vi "模块参数配置.vi"(9 "路径":path, 10 "历史中心参数2":T2={"IP地址"="192.168.1.1", "工作模式"=48, "连接协议"=48, "本机号码"="13806871122", "短信监控中心号码1"="13800577500", "监听时间"=0, "心跳间隔"=0, "重启时间(分)"=0, "C/S关系"=48, "DNS域名"="", "APN接入点"="", "报头使能"=48, "波特率"=45060, "短信目标号码1 "="", "短信目标号码2"="", "短信监控中心号码2"="", "信号检测使能"=48, "控制方式"=48, "端口号"=5070, "连接方式"=48} {"连接方式" items=["固定IP"=48, "域名解析"=49]; "控制方式" items=["软件控制"=48, "EN控制"=49]; "信号检测使能" items=["不检测"=48, "检测"=49]; "波特率" items=["1200"=45060, "2400"=24585, "4800"=49170, "9600"=32805, "19200"=75]; "报头使能" items=["上传"=48, "不上传"=49]; "C/S关系" items=["客服端"=48, "服务端"=49]; "连接协议" items=["TCP协议"=48, "UDP协议"=49]; "工作模式" items=["GPRS模式"=48, "短信模式"=49]}, 11 "历史中心参数1":T2={"IP地址"="192.168.1.1", "工作模式"=48, "连接协议"=48, "本机号码"="13806871122", "短信监控中心号码1"="13800577500", "监听时间"=0, "心跳间隔"=0, "重启时间(分)"=0, "C/S关系"=48, "DNS域名"="", "APN接入点"="", "报头使能"=48, "波特率"=45060, "短信目标号码1 "="", "短信目标号码2"="", "短信监控中心号码2"="", "信号检测使能"=48, "控制方式"=48, "端口号"=5070, "连接方式"=48} {"连接方式" items=["固定IP"=48, "域名解析"=49]; "控制方式" items=["软件控制"=48, "EN控制"=49]; "信号检测使能" items=["不检测"=48, "检测"=49]; "波特率" items=["1200"=45060, "2400"=24585, "4800"=49170, "9600"=32805, "19200"=75]; "报头使能" items=["上传"=48, "不上传"=49]; "C/S关系" items=["客服端"=48, "服务端"=49]; "连接协议" items=["TCP协议"=48, "UDP协议"=49]; "工作模式" items=["GPRS模式"=48, "短信模式"=49]}) -> ()   [LabVIEW 2015]
uses:
  <vilib>/Utility/config.llb/Config Data RefNum.ctl
  <vilib>/Utility/config.llb/Write Key (String).vi
  <vilib>/Utility/config.llb/NI_LVConfig.lvlib
panel:
  out "输出配置文件":T1 caption="refnum out"
  out "保存参数数组":bool[](array[boolean])
  out "读参数数组":bool[](array[boolean])
  out "写参数数组":bool[](array[boolean])
  out "复制数组":bool[](array[boolean])
  in  "》2":bool
  in  "》1":bool
  in  "模块中心参数2":T2={"IP地址"="192.168.1.1", "工作模式"=48, "连接协议"=48, "本机号码"="13806871122", "短信监控中心号码1"="13800577500", "监听时间"=0, "心跳间隔"=0, "重启时间(分)"=0, "C/S关系"=48, "DNS域名"="", "APN接入点"="", "报头使能"=48, "波特率"=45060, "短信目标号码1 "="", "短信目标号码2"="", "短信监控中心号码2"="", "信号检测使能"=48, "控制方式"=48, "端口号"=5070, "连接方式"=48} {"连接方式" items=["固定IP"=48, "域名解析"=49]; "控制方式" items=["软件控制"=48, "EN控制"=49]; "信号检测使能" items=["不检测"=48, "检测"=49]; "波特率" items=["1200"=45060, "2400"=24585, "4800"=49170, "9600"=32805, "19200"=75]; "报头使能" items=["上传"=48, "不上传"=49]; "C/S关系" items=["客服端"=48, "服务端"=49]; "连接协议" items=["TCP协议"=48, "UDP协议"=49]; "工作模式" items=["GPRS模式"=48, "短信模式"=49]}
  in  "模块中心参数1":T2={"IP地址"="192.168.1.1", "工作模式"=48, "连接协议"=48, "本机号码"="13806871122", "短信监控中心号码1"="13800577500", "监听时间"=0, "心跳间隔"=0, "重启时间(分)"=0, "C/S关系"=48, "DNS域名"="", "APN接入点"="", "报头使能"=48, "波特率"=45060, "短信目标号码1 "="", "短信目标号码2"="", "短信监控中心号码2"="", "信号检测使能"=48, "控制方式"=48, "端口号"=5070, "连接方式"=48} {"连接方式" items=["固定IP"=48, "域名解析"=49]; "控制方式" items=["软件控制"=48, "EN控制"=49]; "信号检测使能" items=["不检测"=48, "检测"=49]; "波特率" items=["1200"=45060, "2400"=24585, "4800"=49170, "9600"=32805, "19200"=75]; "报头使能" items=["上传"=48, "不上传"=49]; "C/S关系" items=["客服端"=48, "服务端"=49]; "连接协议" items=["TCP协议"=48, "UDP协议"=49]; "工作模式" items=["GPRS模式"=48, "短信模式"=49]}
  in  "写入模块参数二":bool
  in  "写入模块参数一":bool
  in  "保存历史参数二":bool
  in  "保存历史参数一":bool
  in  "获取模块参数二":bool
  in  "获取模块参数一":bool
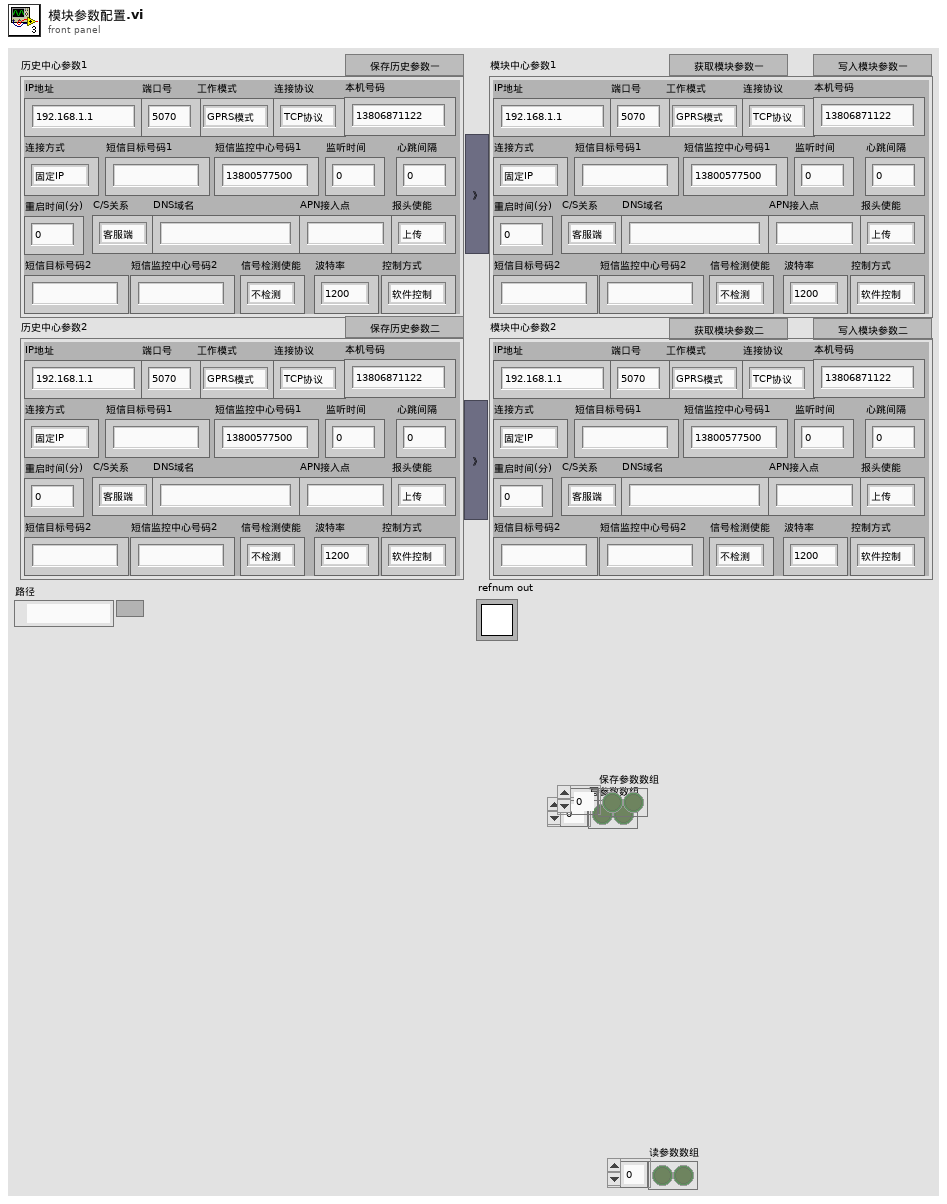
[diagram p1: front panel]
types:
  T1 = typedef "NI_LVConfig.lvlib/Config Data RefNum.ctl" = refnum<k1>
  T2 = typedef "GPRS参数DW02.ctl" = cluster{"IP地址":string, "工作模式":u16, "连接协议":u16, "本机号码":string, "短信监控中心号码1":string, "监听时间":u16, "心跳间隔":u16, "重启时间(分)":u16, "C/S关系":u16, "DNS域名":string, "APN接入点":string, "报头使能":u16, "波特率":u16, "短信目标号码1 ":string, "短信目标号码2":string, "短信监控中心号码2":string, "信号检测使能":u16, "控制方式":u16, "端口号":u16, "连接方式":u16}
  T3 = typedef "模块参数配置状态机状态(枚举).ctl" = enum16{"初始化", "加载参数", "等待按键", "写参数", "读参数", "拷贝参数", "保存参数", "退出"}
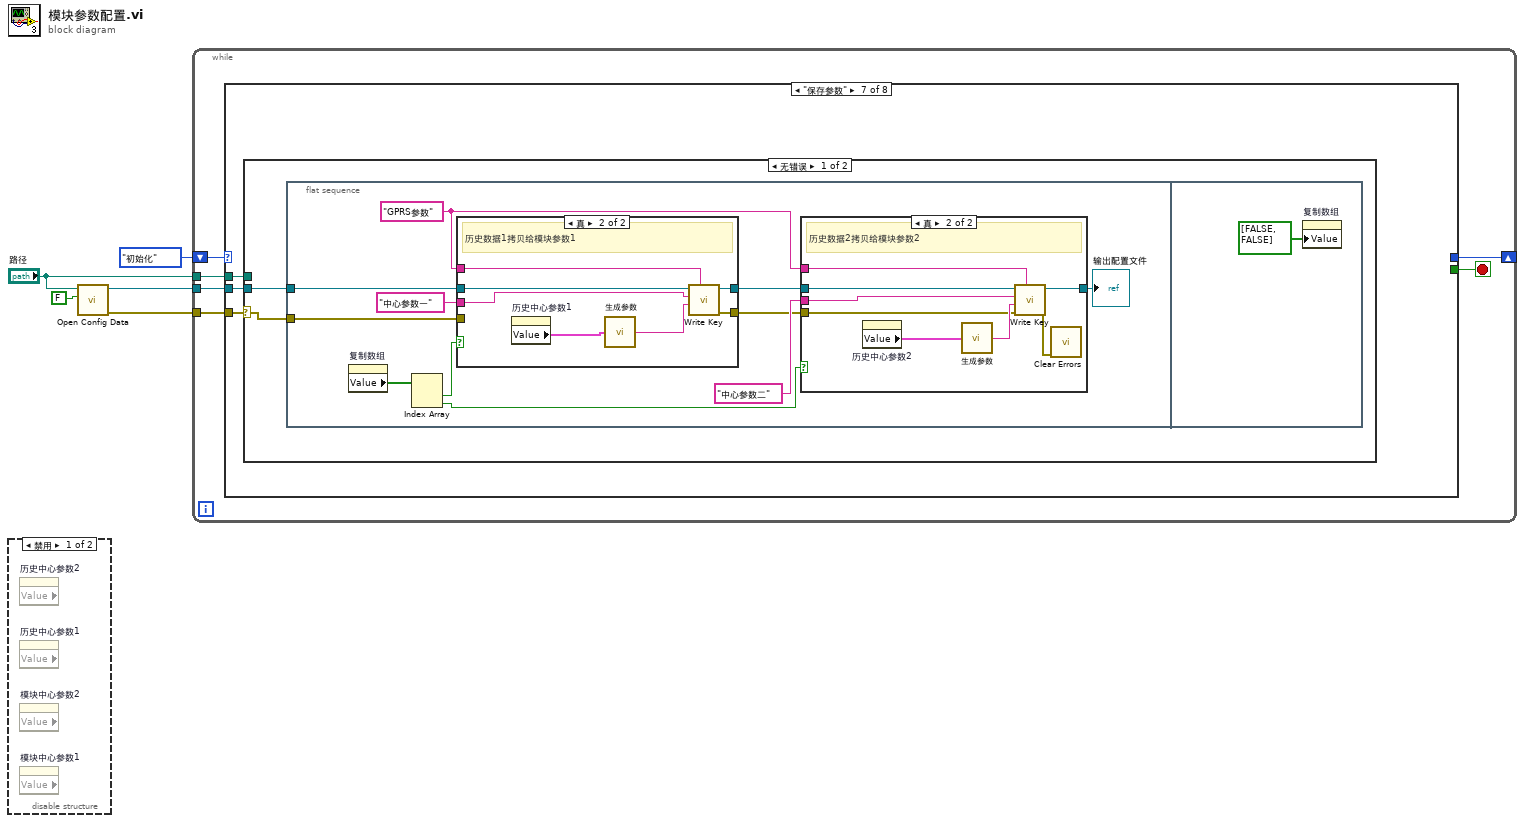
[diagram p0: block diagram]
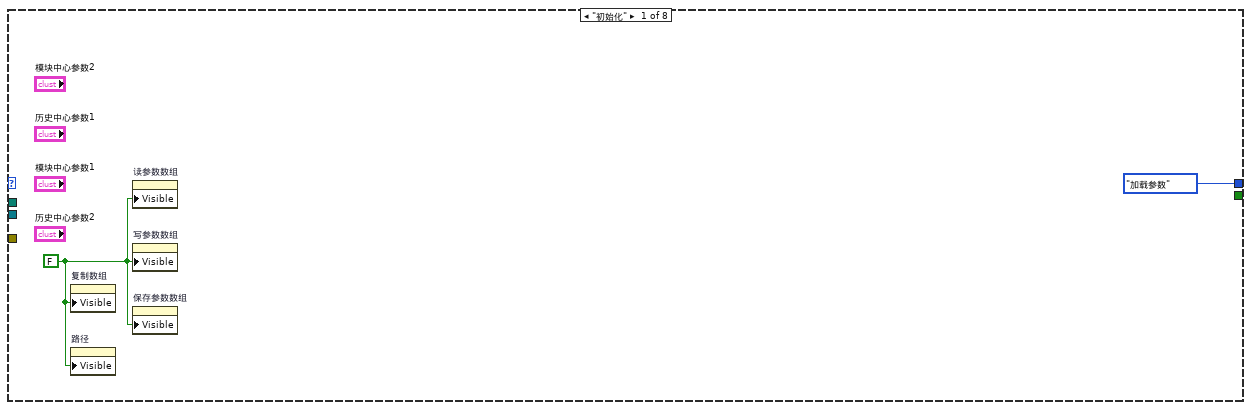
[diagram p3: hidden frame]
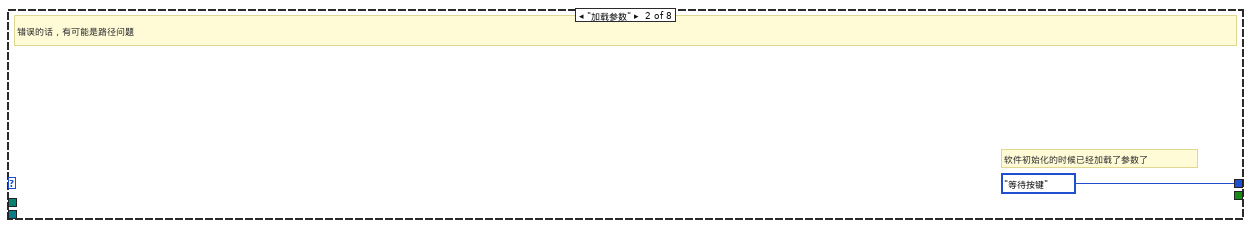
[diagram p4: hidden frame]
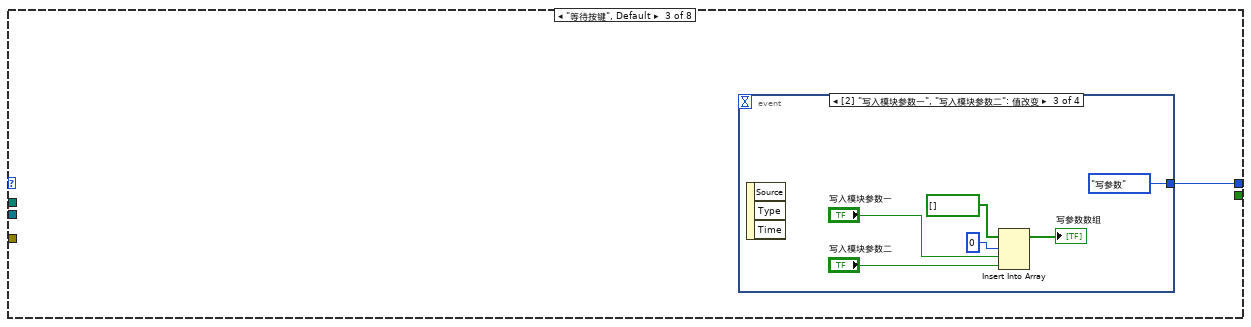
[diagram p5: hidden frame]
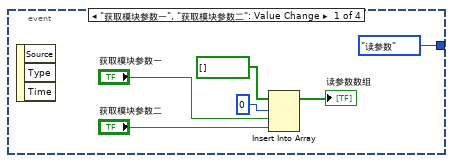
[diagram p6: hidden frame]
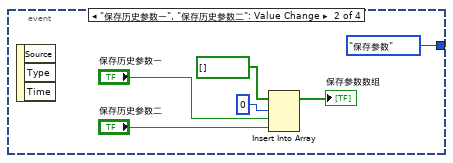
[diagram p7: hidden frame]
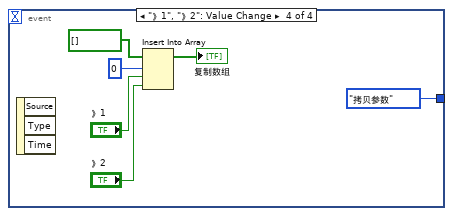
[diagram p8: hidden frame]
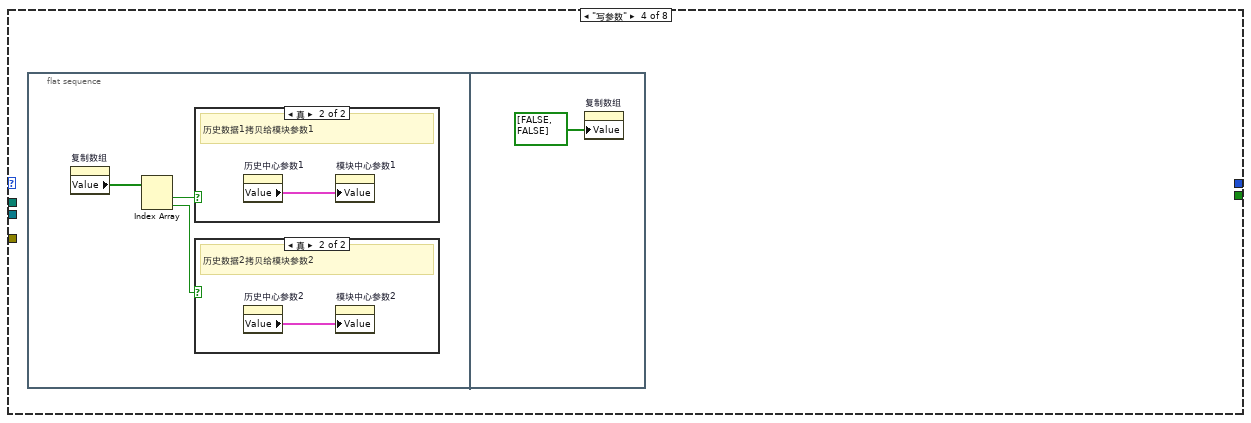
[diagram p9: hidden frame]
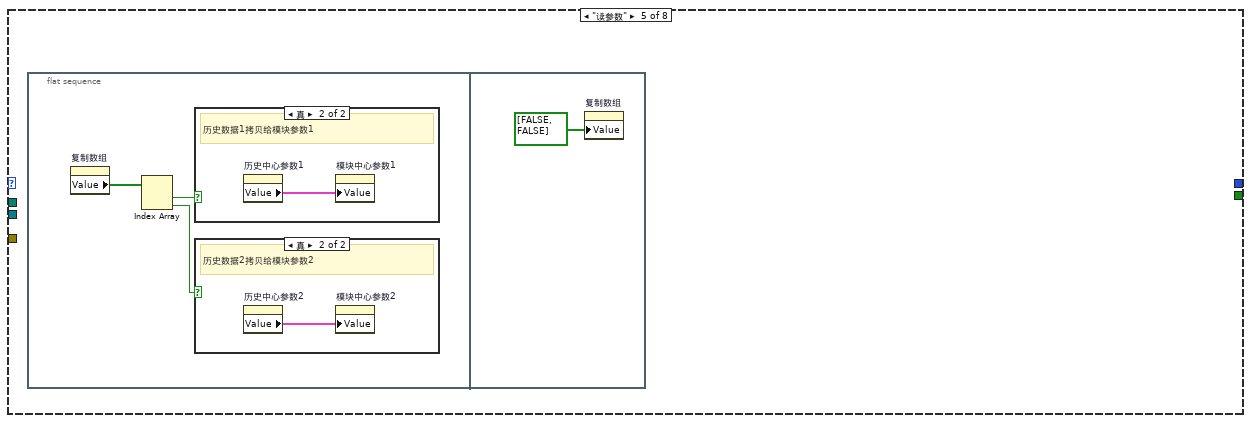
[diagram p12: hidden frame]
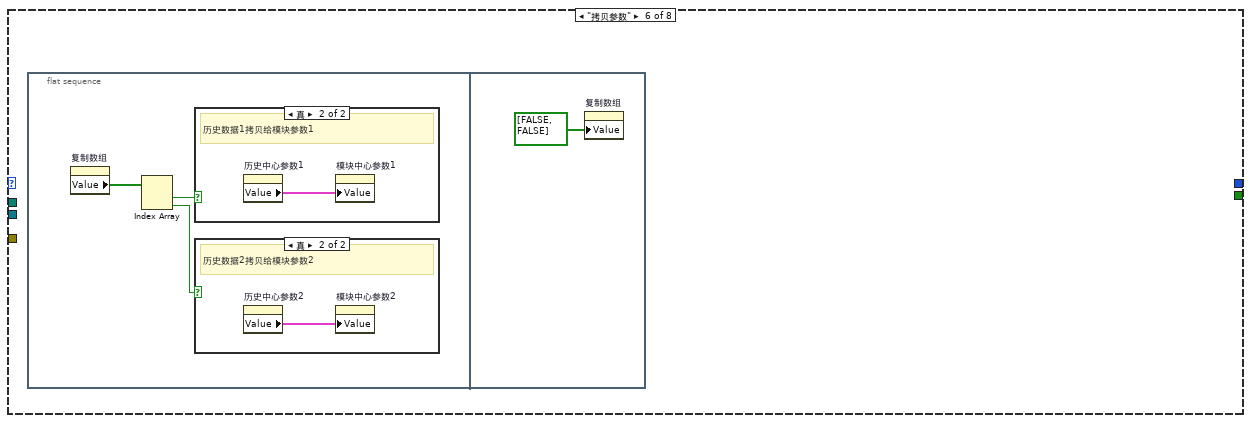
[diagram p15: hidden frame]
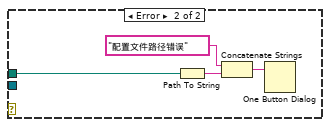
[diagram p20: hidden frame]
diagram:
  n1 = disable-structure shown="禁用" {
    frame Disabled {
      n2 = property on="历史中心参数2" class="Clust (严格)" props=["Value"]() -> ()  [unwired: 2 in, 3 out]
      n3 = property on="历史中心参数1" class="Clust (严格)" props=["Value"]() -> ()  [unwired: 2 in, 3 out]
      n4 = property on="模块中心参数2" class="Clust (严格)" props=["Value"]() -> ()  [unwired: 2 in, 3 out]
      n5 = property on="模块中心参数1" class="Clust (严格)" props=["Value"]() -> ()  [unwired: 2 in, 3 out]
    }
    frame Enabled {
    }
  }
  n6 = call <vilib>:"Open Config Data.vi"("create file if necessary (T)"=FALSE, "configuration file path"="路径") -> ("error out"=w2:errorcluster, "refnum"=w3:T1)  [unwired: 7 in, 1 out]
  n7 = while {
    shift-right: [w10] -> _
    shift-left: 模块参数配置状态机状态(枚举)."初始化" -> [w9]
    tunnel: w3 -> [w8]
    tunnel: w2 -> [w7]
    tunnel: "路径" -> [w6]
    stop <- w11 stop-if-true
    n8 = case shown="\"保存参数\"" w9 {
      tunnel: [_ _ _ _ _ _ _ TRUE] -> w11
      tunnel: [模块参数配置状态机状态(枚举)."加载参数" 模块参数配置状态机状态(枚举)."等待按键" w15 _ _ _ _ _] -> w10
      tunnel: w8 -> [_ _ _ _ _ _ w60 _]
      tunnel: w7 -> [_ _ _ _ _ _ w59 _]
      tunnel: w6 -> [_ _ _ _ _ _ w58 _]
      frame "初始化" {
        w12 = FALSE ("可见")
        n9 = property on="复制数组" class="Arr (严格)"("Visible"=w12) -> ()  [unwired: 2 in, 2 out]
        n10 = property on="路径" class="Path"("Visible"=w12) -> ()  [unwired: 2 in, 2 out]
        n11 = property on="读参数数组" class="Arr (严格)"("Visible"=w12) -> ()  [unwired: 2 in, 2 out]
        n12 = property on="写参数数组" class="Arr (严格)"("Visible"=w12) -> ()  [unwired: 2 in, 2 out]
        n13 = property on="保存参数数组" class="Arr (严格)"("Visible"=w12) -> ()  [unwired: 2 in, 2 out]
      }
      frame "加载参数" {
        # "软件初始化的时候已经加载了参数了"
        # "错误的话，有可能是路径问题"
      }
      frame "等待按键", Default {
        n14 = event shown="[2] \"写入模块参数一\", \"写入模块参数二\": 值改变" {
          selector: _ -> [_ _ _ _]
          dyn-events: _ -> [_ _ _ _]
          timeout: _ -> [_ _ _ _]
          tunnel: [模块参数配置状态机状态(枚举)."读参数" 模块参数配置状态机状态(枚举)."保存参数" 模块参数配置状态机状态(枚举)."写参数" 模块参数配置状态机状态(枚举)."拷贝参数"] -> w15
          event "获取模块参数一", "获取模块参数二": Value Change {
            n15 = event-data() -> ()  [unwired: 1 in, 3 out]
            n16 = Insert Into Array(array=bool[] [] ("数组"), index=0 ("索引"), new element #1="获取模块参数一", new element #2="获取模块参数二") -> (→"读参数数组":bool[])
          }
          event "保存历史参数一", "保存历史参数二": Value Change {
            n17 = event-data() -> ()  [unwired: 1 in, 3 out]
            n18 = Insert Into Array(array=bool[] [] ("数组"), index=0 ("索引"), new element #1="保存历史参数一", new element #2="保存历史参数二") -> (→"保存参数数组":bool[])
          }
          event "写入模块参数一", "写入模块参数二": Value Change {
            n19 = event-data() -> ()  [unwired: 1 in, 3 out]
            n20 = Insert Into Array(array=bool[] [] ("数组"), index=0 ("索引"), new element #1="写入模块参数一", new element #2="写入模块参数二") -> (→"写参数数组":bool[])
          }
          event "》1", "》2": Value Change {
            n21 = event-data() -> ()  [unwired: 1 in, 3 out]
            n22 = Insert Into Array(array=bool[] [] ("数组"), index=0 ("索引"), new element #1="》1", new element #2="》2") -> (→"复制数组":bool[])
          }
        }
      }
      frame "写参数" {
        n23 = flat-sequence {
          frame #0 {
            n24 = property on="复制数组" class="Arr (严格)"() -> ("Value"=w42:bool[])  [unwired: 2 in, 2 out]
            n25 = Index Array(array=w42) -> (element #1=w41:bool, element #2=w40:bool)  [unwired: 2 in]
            n26 = case shown="真" w41 {
              frame False {
              }
              frame True {
                # "历史数据1拷贝给模块参数1"
                n27 = property on="历史中心参数1" class="Clust (严格)"() -> ("Value"=w44:T2)  [unwired: 2 in, 2 out]
                n28 = property on="模块中心参数1" class="Clust (严格)"("Value"=w44) -> ()  [unwired: 2 in, 2 out]
              }
            }
            n29 = case shown="真" w40 {
              frame False {
              }
              frame True {
                # "历史数据2拷贝给模块参数2"
                n30 = property on="历史中心参数2" class="Clust (严格)"() -> ("Value"=w43:T2)  [unwired: 2 in, 2 out]
                n31 = property on="模块中心参数2" class="Clust (严格)"("Value"=w43) -> ()  [unwired: 2 in, 2 out]
              }
            }
          }
          frame #1 {
            n32 = property on="复制数组" class="Arr (严格)"("Value"=bool[] [FALSE, FALSE] ("复制数组")) -> ()  [unwired: 2 in, 2 out]
          }
        }
      }
      frame "读参数" {
        n33 = flat-sequence {
          frame #0 {
            n34 = property on="复制数组" class="Arr (严格)"() -> ("Value"=w48:bool[])  [unwired: 2 in, 2 out]
            n35 = Index Array(array=w48) -> (element #1=w47:bool, element #2=w46:bool)  [unwired: 2 in]
            n36 = case shown="真" w47 {
              frame False {
              }
              frame True {
                # "历史数据1拷贝给模块参数1"
                n37 = property on="历史中心参数1" class="Clust (严格)"() -> ("Value"=w50:T2)  [unwired: 2 in, 2 out]
                n38 = property on="模块中心参数1" class="Clust (严格)"("Value"=w50) -> ()  [unwired: 2 in, 2 out]
              }
            }
            n39 = case shown="真" w46 {
              frame False {
              }
              frame True {
                # "历史数据2拷贝给模块参数2"
                n40 = property on="历史中心参数2" class="Clust (严格)"() -> ("Value"=w49:T2)  [unwired: 2 in, 2 out]
                n41 = property on="模块中心参数2" class="Clust (严格)"("Value"=w49) -> ()  [unwired: 2 in, 2 out]
              }
            }
          }
          frame #1 {
            n42 = property on="复制数组" class="Arr (严格)"("Value"=bool[] [FALSE, FALSE] ("复制数组")) -> ()  [unwired: 2 in, 2 out]
          }
        }
      }
      frame "拷贝参数" {
        n43 = flat-sequence {
          frame #0 {
            n44 = property on="复制数组" class="Arr (严格)"() -> ("Value"=w54:bool[])  [unwired: 2 in, 2 out]
            n45 = Index Array(array=w54) -> (element #1=w53:bool, element #2=w52:bool)  [unwired: 2 in]
            n46 = case shown="真" w53 {
              frame False {
              }
              frame True {
                # "历史数据1拷贝给模块参数1"
                n47 = property on="历史中心参数1" class="Clust (严格)"() -> ("Value"=w56:T2)  [unwired: 2 in, 2 out]
                n48 = property on="模块中心参数1" class="Clust (严格)"("Value"=w56) -> ()  [unwired: 2 in, 2 out]
              }
            }
            n49 = case shown="真" w52 {
              frame False {
              }
              frame True {
                # "历史数据2拷贝给模块参数2"
                n50 = property on="历史中心参数2" class="Clust (严格)"() -> ("Value"=w55:T2)  [unwired: 2 in, 2 out]
                n51 = property on="模块中心参数2" class="Clust (严格)"("Value"=w55) -> ()  [unwired: 2 in, 2 out]
              }
            }
          }
          frame #1 {
            n52 = property on="复制数组" class="Arr (严格)"("Value"=bool[] [FALSE, FALSE] ("复制数组")) -> ()  [unwired: 2 in, 2 out]
          }
        }
      }
      frame "保存参数" {
        n53 = case shown="无错误" w59 {
          selector: w59 -> [w61 _]
          tunnel: w60 -> [w62 _]
          tunnel: w58 -> [_ w96]
          frame No Error {
            n54 = flat-sequence {
              tunnel: w62 -> [w67]
              tunnel: w61 -> [w63]
              frame #0 {
                w69 = "GPRS参数" ("section")
                n55 = property on="复制数组" class="Arr (严格)"() -> ("Value"=w73:bool[])  [unwired: 2 in, 2 out]
                n56 = Index Array(array=w73) -> (element #1=w72:bool, element #2=w71:bool)  [unwired: 2 in]
                n57 = case shown="真" w72 {
                  tunnel: w67 -> [w84 w90]
                  tunnel: "中心参数一" ("section") -> [_ w89]
                  tunnel: w69 -> [_ w88]
                  tunnel: [w84 w86] -> w66
                  tunnel: [w83 w85] -> w64
                  tunnel: w63 -> [w83 _]
                  frame False {
                  }
                  frame True {
                    # "历史数据1拷贝给模块参数1"
                    n58 = property on="历史中心参数1" class="Clust (严格)"() -> ("Value"=w91:T2)  [unwired: 2 in, 2 out]
                    n59 = call "生成参数.vi"("GPRS参数（TXJT）"=w91) -> ("字符串"=w87:string)
                    n60 = call-poly <vilib>:"Write Key.vi"("section"=w88, "value"=w87, "key"=w89, "refnum"=w90) -> ("error out"=w85:errorcluster, "refnum out"=w86:T1)  [unwired: 5 in, 1 out]
                  }
                }
                n61 = case shown="真" w71 {
                  tunnel: w69 -> [_ w81]
                  tunnel: "中心参数二" ("section") -> [_ w80]
                  tunnel: w66 -> [w74 w79]
                  tunnel: [w74 w77] -> w65
                  tunnel: w64 -> [_ w75]
                  frame False {
                  }
                  frame True {
                    # "历史数据2拷贝给模块参数2"
                    n62 = property on="历史中心参数2" class="Clust (严格)"() -> ("Value"=w82:T2)  [unwired: 2 in, 2 out]
                    n63 = call "生成参数.vi"("GPRS参数（TXJT）"=w82) -> ("字符串"=w78:string)
                    n64 = call-poly <vilib>:"Write Key.vi"("section"=w81, "error in (no error)"=w75, "value"=w78, "key"=w80, "refnum"=w79) -> ("error out"=w76:errorcluster, "refnum out"=w77:T1)  [unwired: 4 in, 1 out]
                    n65 = call <vilib>:"Clear Errors.vi"("error in (no error)"=w76) -> ()  [unwired: 5 in, 2 out]
                  }
                }
                "输出配置文件" <- w65
              }
              frame #1 {
                n66 = property on="复制数组" class="Arr (严格)"("Value"=bool[] [FALSE, FALSE] ("复制数组")) -> ()  [unwired: 2 in, 2 out]
              }
            }
          }
          frame Error {
            n67 = Path To String(path=w96) -> (string=w95:string)
            n68 = Concatenate Strings("配置文件路径错误" ("消息"), w95) -> (w93:string)
            n69 = One Button Dialog(message=w93) -> ()  [unwired: 1 in, 1 out]
          }
        }
      }
      frame "退出" {
        n70 = property on="输出配置文件" class="TypRef (严格)"() -> (error out=w98:errorcluster, "Value"=w99:T1)  [unwired: 2 in, 1 out]
        n71 = call <vilib>:"Close Config Data.vi"("error in (no error)"=w98, "refnum"=w99) -> ("error out"=w97:errorcluster)  [unwired: 8 in, 1 out]
        n72 = call <vilib>:"Clear Errors.vi"("error in (no error)"=w97) -> ()  [unwired: 5 in, 2 out]
      }
    }
  }
